vi "html waiting.vi"(8 "error in (no error)":errorcluster, 11 "WebView2 Control":refnum<vi>) -> (0 "error out":errorcluster)   [LabVIEW 2020, in "splash_screen.lvclass"]
uses:
  splash_screen.lvclass
  <vilib>/sklein/WebView2/Webview2 Control/WebView2 Control.xctl
  <vilib>/sklein/WebView2/Webview2 Control/Paths.ctl
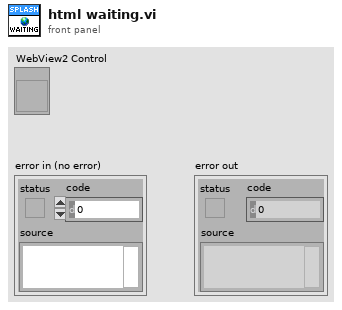
[diagram p1: front panel]
types:
  T1 = typedef "WebView2 Control.xctl/Paths.ctl" = cluster{"Webview2 Native":path, "Edge Application":path, "User Data":path}
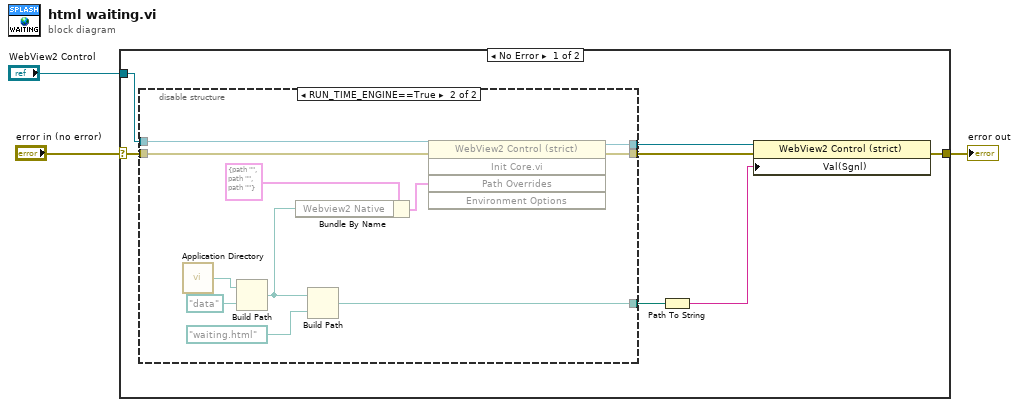
[diagram p0: block diagram]
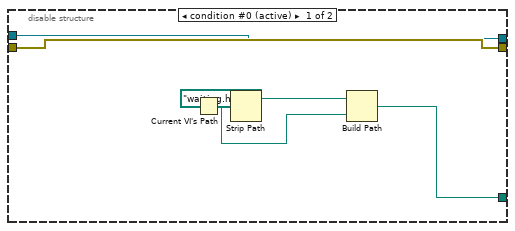
[diagram p2: hidden frame]
diagram:
  n1 = case shown="No Error" "error in (no error)" {
    selector: "error in (no error)" -> [w7 w28]
    tunnel: [w5 w28] -> w2
    tunnel: "WebView2 Control" -> [w8 _]
    frame No Error {
      n2 = disable-structure shown="RUN_TIME_ENGINE==True" {
        disable-tunnel: [w15 w25] -> w10
        disable-tunnel: [w12 w21] -> w6
        disable-tunnel: w7 -> [w12 w22]
        disable-tunnel: w8 -> [w11 w18]
        disable-tunnel: [w11 w17] -> w4
        frame condition #0 (active) {
          n3 = Current VI's Path() -> (path=w16:path)
          n4 = Strip Path(path=w16) -> (stripped path=w13:path)  [unwired: 1 out]
          n5 = Build Path(base path=w13, name or relative path=path "waiting.html") -> (appended path=w15:path)
        }
        frame condition #1 {
          n6 = call <vilib>:"Application Directory.vi"() -> ("Application Directory"=w27:path)
          n7 = Build Path(base path=w27, name or relative path=path "data") -> (appended path=w19:path)
          n8 = Bundle By Name(cluster=T1 {"Webview2 Native"=path "", "Edge Application"=path "", "User Data"=path ""} ("Path Overrides"), "Webview2 Native"=w19) -> (w20:T1)
          n9 = Build Path(base path=w19, name or relative path=path "waiting.html") -> (appended path=w25:path)
          n10 = invoke on="Invoke Node" class="WebView2 Control (strict)" method="Init Core.vi"(reference=w18, error in=w22, "Path Overrides"=w20) -> (reference out=w17:refnum<vi>, error out=w21:errorcluster)  [unwired: 2 in, 3 out]
        }
      }
      n11 = Path To String(path=w10) -> (string=w9:string)
      n12 = property on="Property Node" class="WebView2 Control (strict)"(reference=w4, error in=w6, "Val(Sgnl)"=w9) -> (error out=w5:errorcluster)  [unwired: 1 out]
    }
    frame Error {
    }
  }
  "error out" <- w2
